vi "Position.vi"(8 "error in (no error)":errorcluster, 10 "Panel VI":refnum<vi>, 11 "Reference Position in":refnum<class "Reference Position.lvclass">) -> (0 "error out":errorcluster, 2 "Open Maximized?":bool)   [LabVIEW 2023, in "Panel Actor.lvlib" / "Panel.lvlib" / "Reference Position.lvclass"]
doc: "Positions the panel based on the reference rectangle and aligment info.\n\n----\nPlease see the following web address for additional documentation and tutorial information:\nhttp://www.mooregoodideas.com/mgi-panel-manager/\n\nAuthor: Derek Trepanier\n\nCopyright (c) 2018, Moore Good Ideas, Inc.\n\nAll rights reserved.\n\nRedistribution and use in source and binary forms, with or without modification, are permitted provided that the following conditions are met:\n\n * Redistributions of source code must retain the above copyright notice, this list of conditions and the following disclaimer.\n * Redistributions in binary form must reproduce the above copyright notice, this list of conditions and the following disclaimer in the documentation and/or other materials provided with the distribution.\n * Neither the name of Moore Good Ideas, Inc. nor the names of its contributors may be used to endorse or promote products derived from this software without specific prior written permission.\n\nTHIS SOFTWARE IS PROVIDED BY THE COPYRIGHT HOLDERS AND CONTRIBUTORS \"AS IS\" AND ANY EXPRESS OR IMPLIED WARRANTIES, INCLUDING, BUT NOT LIMITED TO, THE IMPLIED WARRANTIES OF MERCHANTABILITY AND FITNESS FOR A PARTICULAR PURPOSE ARE DISCLAIMED. IN NO EVENT SHALL THE COPYRIGHT OWNER OR CONTRIBUTORS BE LIABLE FOR ANY DIRECT, INDIRECT, INCIDENTAL, SPECIAL, EXEMPLARY, OR CONSEQUENTIAL DAMAGES (INCLUDING, BUT NOT LIMITED TO, PROCUREMENT OF SUBSTITUTE GOODS OR SERVICES; LOSS OF USE, DATA, OR PROFITS; OR BUSINESS INTERRUPTION) HOWEVER CAUSED AND ON ANY THEORY OF LIABILITY, WHETHER IN CONTRACT, STRICT LIABILITY, OR TORT (INCLUDING NEGLIGENCE OR OTHERWISE) ARISING IN ANY WAY OUT OF THE USE OF THIS SOFTWARE, EVEN IF ADVISED OF THE POSSIBILITY OF SUCH DAMAGE."
uses:
  Reference Position.lvclass
  Reference Position.lvclass/Reference Position.ctl
  <vilib>/Utility/miscctls.llb/LVRectTypeDef.ctl
  Size/Size.lvclass
  Offset/Offset.lvclass
  Panel.lvlib
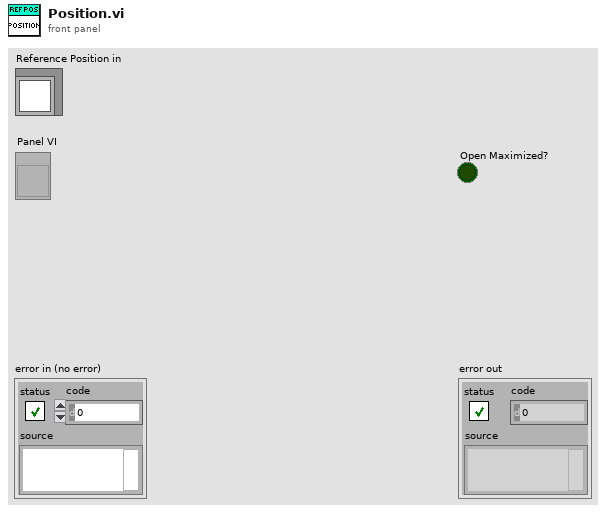
[diagram p1: front panel]
types:
  T1 = cluster{"left":i16, "top":i16, "right":i16, "bottom":i16}
  T2 = cluster{"left":bool, "top":bool, "right":bool, "bottom":bool}
  T3 = typedef "LVRectTypeDef.ctl" = cluster{"Left":i16, "Top":i16, "Right":i16, "Bottom":i16}
  T4 = typedef "LVPointTypeDef.ctl" = cluster{"Horizontal":i16, "Vertical":i16}
  T5 = typedef "Panel Actor.lvlib/Panel.lvlib/Reference Position.lvclass/Horizontal Alignment.ctl" = enum16{"Left", "Center", "Right"}
  T6 = typedef "Panel Actor.lvlib/Panel.lvlib/Reference Position.lvclass/Vertical Alignment.ctl" = enum16{"Top", "Center", "Bottom"}
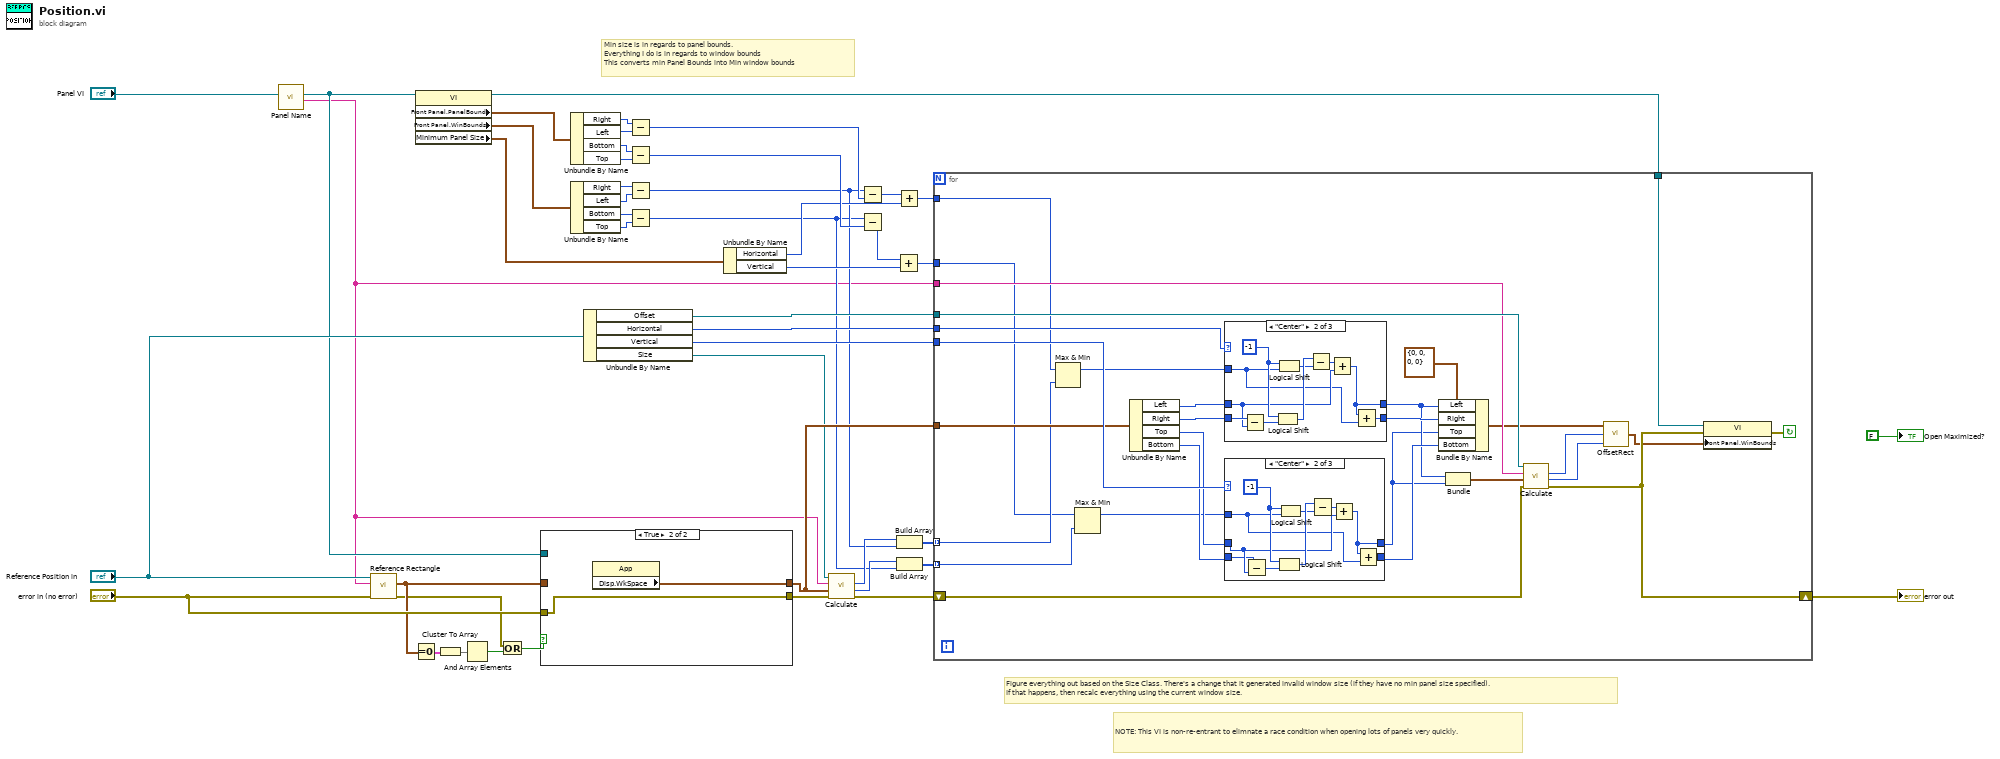
[diagram p0: block diagram]
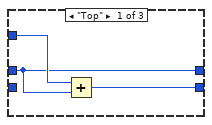
[diagram p2: hidden frame]
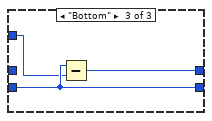
[diagram p3: hidden frame]
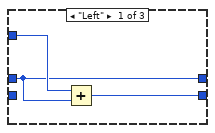
[diagram p4: hidden frame]
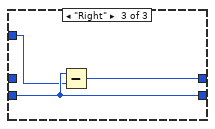
[diagram p5: hidden frame]
diagram:
  # "NOTE: This VI is non-re-entrant to elimnate a race condition when opening lots of panels very quickly."
  # "Figure everything out based on the Size Class. There's a change that it generated invalid window size (if they have no min panel size specified).\nIf that happens, then recalc everything using the current window size."
  # "Min size is in regards to panel bounds.\nEverything I do is in regards to window bounds\nThis converts min Panel Bounds into Min window bounds"
  n1 = call "Panel Name.vi"("VI in"="Panel VI") -> ("Name"=w1:string, "VI out"=w2:refnum<vi>)  [unwired: 9 in]
  n2 = call-dynamic "Reference Rectangle.vi"("error in (no error)"="error in (no error)", "My VI"=w1, "Reference Position in"="Reference Position in") -> ("error out"=w37:errorcluster, "Rectangle"=w41:T1)  [unwired: 7 in]
  n3 = Equal To 0?(x=w41) -> (x = 0?=w40:T2)
  n4 = property class="VI"(reference=w2) -> (reference out=w30:refnum<vi>, "Front Panel.PanelBounds"=w19:T3, "Front Panel.WinBounds"=w18:T3, "Minimum Panel Size"=w29:T4)  [unwired: 1 in, 1 out]
  n5 = Cluster To Array(cluster=w40) -> (array=w39:bool[])
  n6 = And Array Elements(Boolean array=w39) -> (logical AND=w38:bool)
  n7 = Or(x=w37, y=w38) -> (x .or. y?=w36:bool)
  n8 = case shown="True" w36 {
    tunnel: w2 -> [_ _]
    tunnel: w41 -> [w48 _]
    tunnel: [w47 w50] -> w34
    tunnel: "error in (no error)" -> [w47 w50]
    tunnel: [w48 w49] -> w32
    frame False {
    }
    frame True {
      n9 = property class="App"() -> ("Disp.WkSpace"=w49:T3)  [unwired: 2 in, 2 out]
    }
  }
  n10 = Unbundle By Name(w19) -> ("Right"=w13:i16, "Left"=w28:i16, "Bottom"=w27:i16, "Top"=w26:i16)
  n11 = Unbundle By Name(w18) -> ("Right"=w22:i16, "Left"=w23:i16, "Bottom"=w24:i16, "Top"=w25:i16)
  n12 = Unbundle By Name("Reference Position in") -> ("Offset"=w35:refnum<class "Offset.lvclass">, "Horizontal"=w43:T5, "Vertical"=w42:T6, "Size"=w31:refnum<class "Size.lvclass">)
  n13 = Subtract(x=w13, y=w28) -> (x-y=w21:i16)
  n14 = Subtract(x=w27, y=w26) -> (x-y=w20:i16)
  n15 = Subtract(x=w22, y=w23) -> (x-y=w5:i16)
  n16 = Subtract(x=w24, y=w25) -> (x-y=w4:i16)
  n17 = Unbundle By Name(w29) -> ("Horizontal"=w17:i16, "Vertical"=w15:i16)
  n18 = call-dynamic "Calculate.vi"("error in (no error)"=w34, "Reference Rectangle"=w32, "My VI"=w1, "Size in"=w31) -> ("error out"=w33:errorcluster, "Height"=w10:i16, "Width"=w11:i16)  [unwired: 5 in]
  n19 = Subtract(x=w5, y=w21) -> (x-y=w7:i16)
  n20 = Subtract(x=w4, y=w20) -> (x-y=w6:i16)
  n21 = Add(x=w6, y=w15) -> (x+y=w14:i16)
  n22 = Add(x=w7, y=w17) -> (x+y=w16:i16)
  n23 = Build Array(w11, w5) -> (w9:i16[])
  n24 = Build Array(w10, w4) -> (w8:i16[])
  n25 = for {
    tunnel: w43 -> [w79]
    tunnel: w42 -> [w75]
    tunnel: w35 -> [w71]
    tunnel: w1 -> [w69]
    tunnel: w32 -> [w68]
    tunnel: w30 -> [w66]
    tunnel: w9 -> [w65] mode=indexing
    tunnel: w8 -> [w63] mode=indexing
    tunnel: w16 -> [w61]
    tunnel: w14 -> [w60]
    shift-right: [w59] -> w12
    shift-left: w33 -> [w70]
    stop <- w58 continue-if-true
    n26 = Max & Min(x=w61, y=w65) -> (max(x,y)=w64:i16)  [unwired: 1 out]
    n27 = Max & Min(x=w60, y=w63) -> (max(x,y)=w62:i16)  [unwired: 1 out]
    n28 = Unbundle By Name(w68) -> ("Left"=w78:i16, "Right"=w77:i16, "Top"=w74:i16, "Bottom"=w73:i16)
    n29 = case shown="\"Center\"" w79 {
      tunnel: w78 -> [w96 w102 _]
      tunnel: w77 -> [_ w108 w111]
      tunnel: w64 -> [w98 w99 w110]
      tunnel: [w96 w100 w109] -> w57
      tunnel: [w97 w101 w111] -> w76
      frame "Left" {
        n30 = Add(x=w98, y=w96) -> (x+y=w97:i16)
      }
      frame "Center" {
        w106 = i16 -1 ("y")
        n31 = Subtract(x=w108, y=w102) -> (x-y=w107:i16)
        n32 = Logical Shift(y=w106, x=w107) -> (x << y=w104:i16)
        n33 = Logical Shift(y=w106, x=w99) -> (x << y=w103:i16)
        n34 = Subtract(x=w104, y=w103) -> (x-y=w105:i16)
        n35 = Add(x=w105, y=w102) -> (x+y=w100:i16)
        n36 = Add(x=w100, y=w99) -> (x+y=w101:i16)
      }
      frame "Right" {
        n37 = Subtract(x=w111, y=w110) -> (x-y=w109:i16)
      }
    }
    n38 = case shown="\"Center\"" w75 {
      tunnel: w74 -> [w80 w87 _]
      tunnel: w73 -> [_ w86 w95]
      tunnel: w62 -> [w82 w84 w94]
      tunnel: [w80 w85 w93] -> w56
      tunnel: [w81 w83 w95] -> w72
      frame "Top" {
        n39 = Add(x=w82, y=w80) -> (x+y=w81:i16)
      }
      frame "Center" {
        w91 = i16 -1 ("y")
        n40 = Subtract(x=w86, y=w87) -> (x-y=w92:i16)
        n41 = Logical Shift(y=w91, x=w92) -> (x << y=w89:i16)
        n42 = Logical Shift(y=w91, x=w84) -> (x << y=w88:i16)
        n43 = Subtract(x=w89, y=w88) -> (x-y=w90:i16)
        n44 = Add(x=w90, y=w87) -> (x+y=w85:i16)
        n45 = Add(x=w85, y=w84) -> (x+y=w83:i16)
      }
      frame "Bottom" {
        n46 = Subtract(x=w95, y=w94) -> (x-y=w93:i16)
      }
    }
    n47 = Bundle By Name(cluster=T3 {"Left"=0, "Top"=0, "Right"=0, "Bottom"=0} ("Front Panel Window:Window Bounds"), "Left"=w57, "Right"=w76, "Top"=w56, "Bottom"=w72) -> (w54:T3)
    n48 = Bundle("Left"=w57, "Top"=w56) -> (w55:cluster{"Left":i16, "Top":i16})  [unwired: 1 in]
    n49 = call-dynamic "Calculate.vi"("error in (no error)"=w70, "Position in"=w55, "My VI"=w69, "Offset in"=w71) -> ("error out"=w59:errorcluster, "Vertical"=w51:i16, "Horizontal"=w52:i16)  [unwired: 5 in]
    n50 = call <vilib>:"OffsetRect.vi"("v"=w51, "h"=w52, "rect"=w54) -> ("offset rect"=w53:T1)
    n51 = property class="VI"(reference=w66, error in=w59, "Front Panel.WinBounds"=w53) -> (error out=w58:errorcluster)  [unwired: 1 out]
  }
  "error out" <- w12
  "Open Maximized?" <- FALSE ("Open Maximized?")
